vi "FlushSink.vi"(8 "error in (no error)":errorcluster, 11 "FileAppender in":refnum<class "FileAppender.lvclass">) -> (0 "error out":errorcluster, 3 "FileAppender out":refnum<class "FileAppender.lvclass">)   [LabVIEW 2026, in "Lumberjack.lvlib" / "FileAppender.lvclass"]
doc: "Override: flush the open log file's OS buffer to disk (Flush File on currentFileRefnum) so already-written statements are durable before this appender acks the flush. Guarded on Not A Refnum, no-op when no file is open."
uses:
  FileAppender.lvclass
  FileAppender.lvclass/FileAppender.ctl
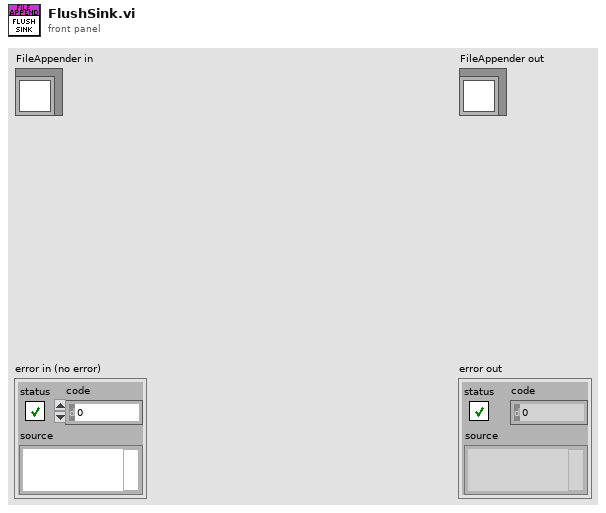
[diagram p1: front panel]
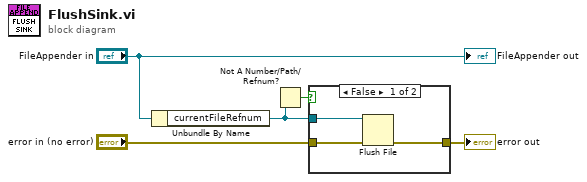
[diagram p0: block diagram]
diagram:
  n1 = Unbundle By Name("FileAppender in") -> ("currentFileRefnum"=w1:refnum<file>)
  n2 = Not A Number/Path/Refnum?(number/path/refnum=w1) -> (NaN/Path/Refnum?=w2:bool)
  n3 = case shown="False" w2 {
    tunnel: w1 -> [w8 _]
    tunnel: "error in (no error)" -> [w7 w9]
    tunnel: [w6 w9] -> w4
    frame False {
      n4 = Flush File(refnum=w8, error in=w7) -> (error out=w6:errorcluster)  [unwired: 1 out]
    }
    frame True {
    }
  }
  "error out" <- w4
  "FileAppender out" <- "FileAppender in"
